vi "FeedBack Chanel.vi"(0 "Test Name":string, 5 "Channels (Int)":i32[](array[numeric]), 7 "FeedBack Channel":string[](array[string])=["fgdgfvcbc", "vnfhgjkn", "21354682"], 9 "Wait/Poll (ms)":u32, 11 "Parameter":u8) -> (4 "Out":i32, 6 "Array":bool[](array[boolean]), 10 "Exit":bool, 12 "Input Status":bool[](array[boolean]), 13 "Channel No":i32[](array[numeric]))   [LabVIEW 2015]
uses:
  Galobal variable_TI.vi
  Project Setup/Globle Variable/GR_Servo.vi
panel:
  out "Result Lvdt":T1
  out "Pokayoka Result":cluster{"Sensor Name":string, "Boolean":bool}[](array[cluster])
  out "output array":bool[](array[boolean])
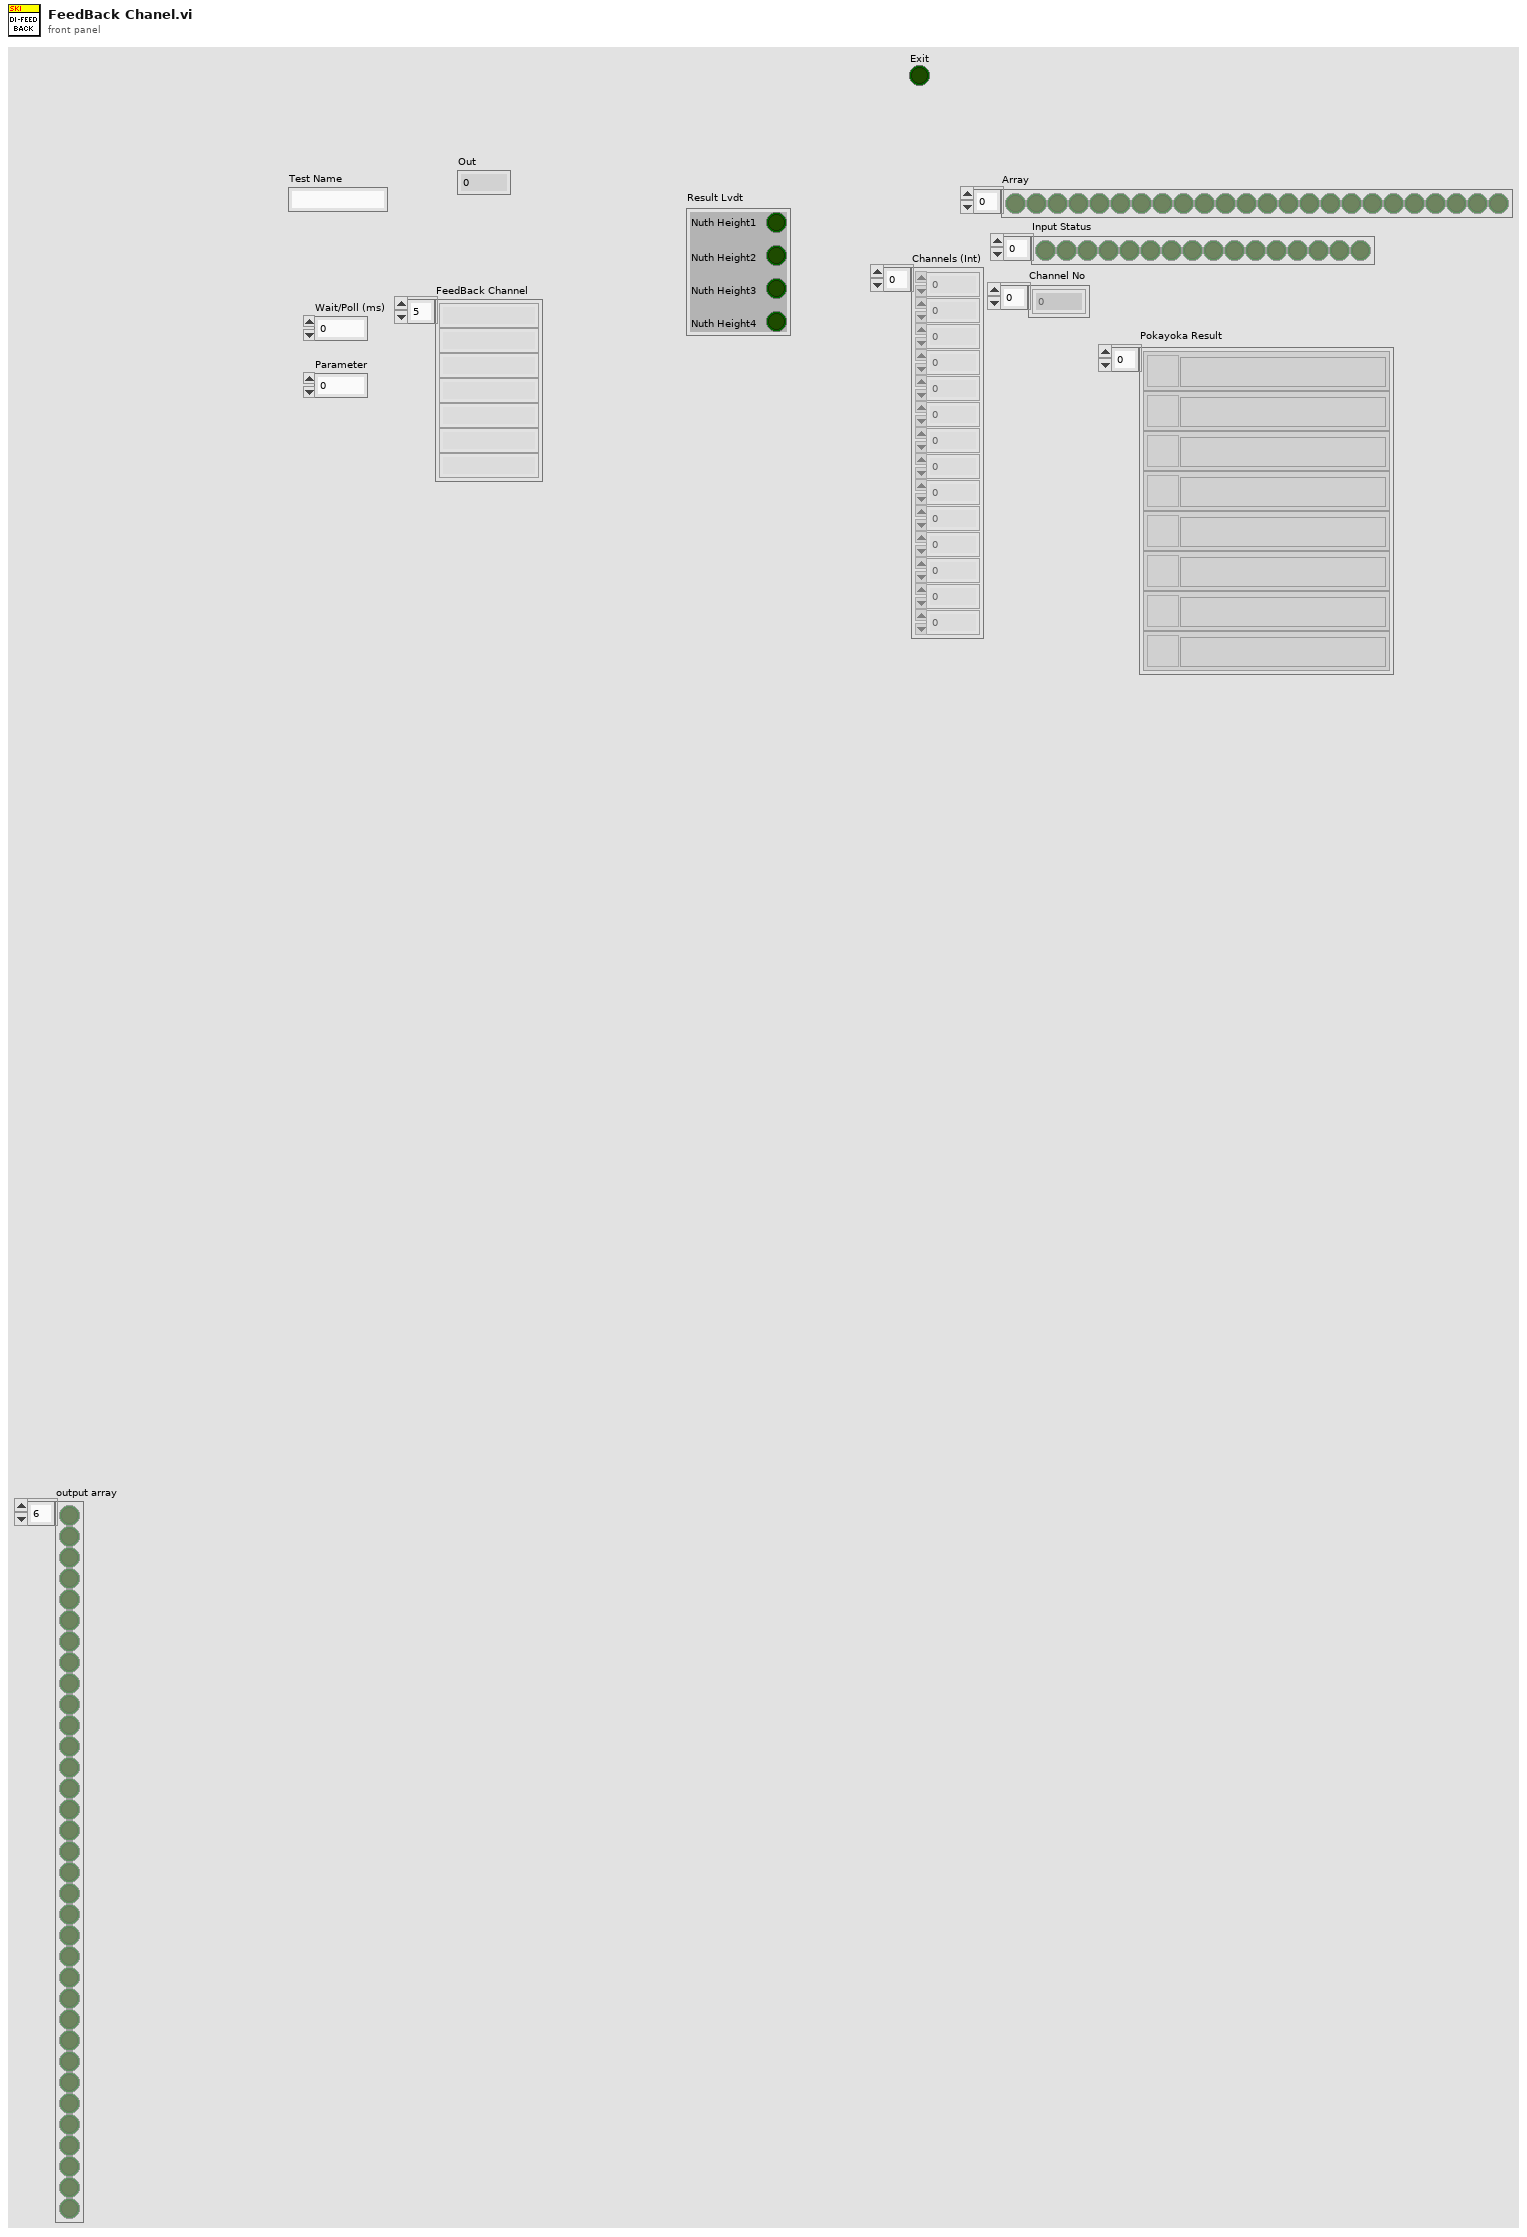
[diagram p1: front panel]
types:
  T1 = cluster{"Nuth Height1":bool, "Nuth Height2":bool, "Nuth Height3":bool, "Nuth Height4":bool}
  T2 = cluster{"LVDT1Max(mm) AI0":dbl, "LVDT1Min (mm)AI0":dbl, "LVDT2Max(mm) AI1":dbl, "LVDT2Min(mm) AI1":dbl, "LVDT3Max(mm) AI2":dbl, "LVDT3Min(mm) AI2":dbl, "LVDT4Max(mm) AI3":dbl, "LVDT4Min(mm) AI3":dbl, "Model":string, "MIC Code":string}
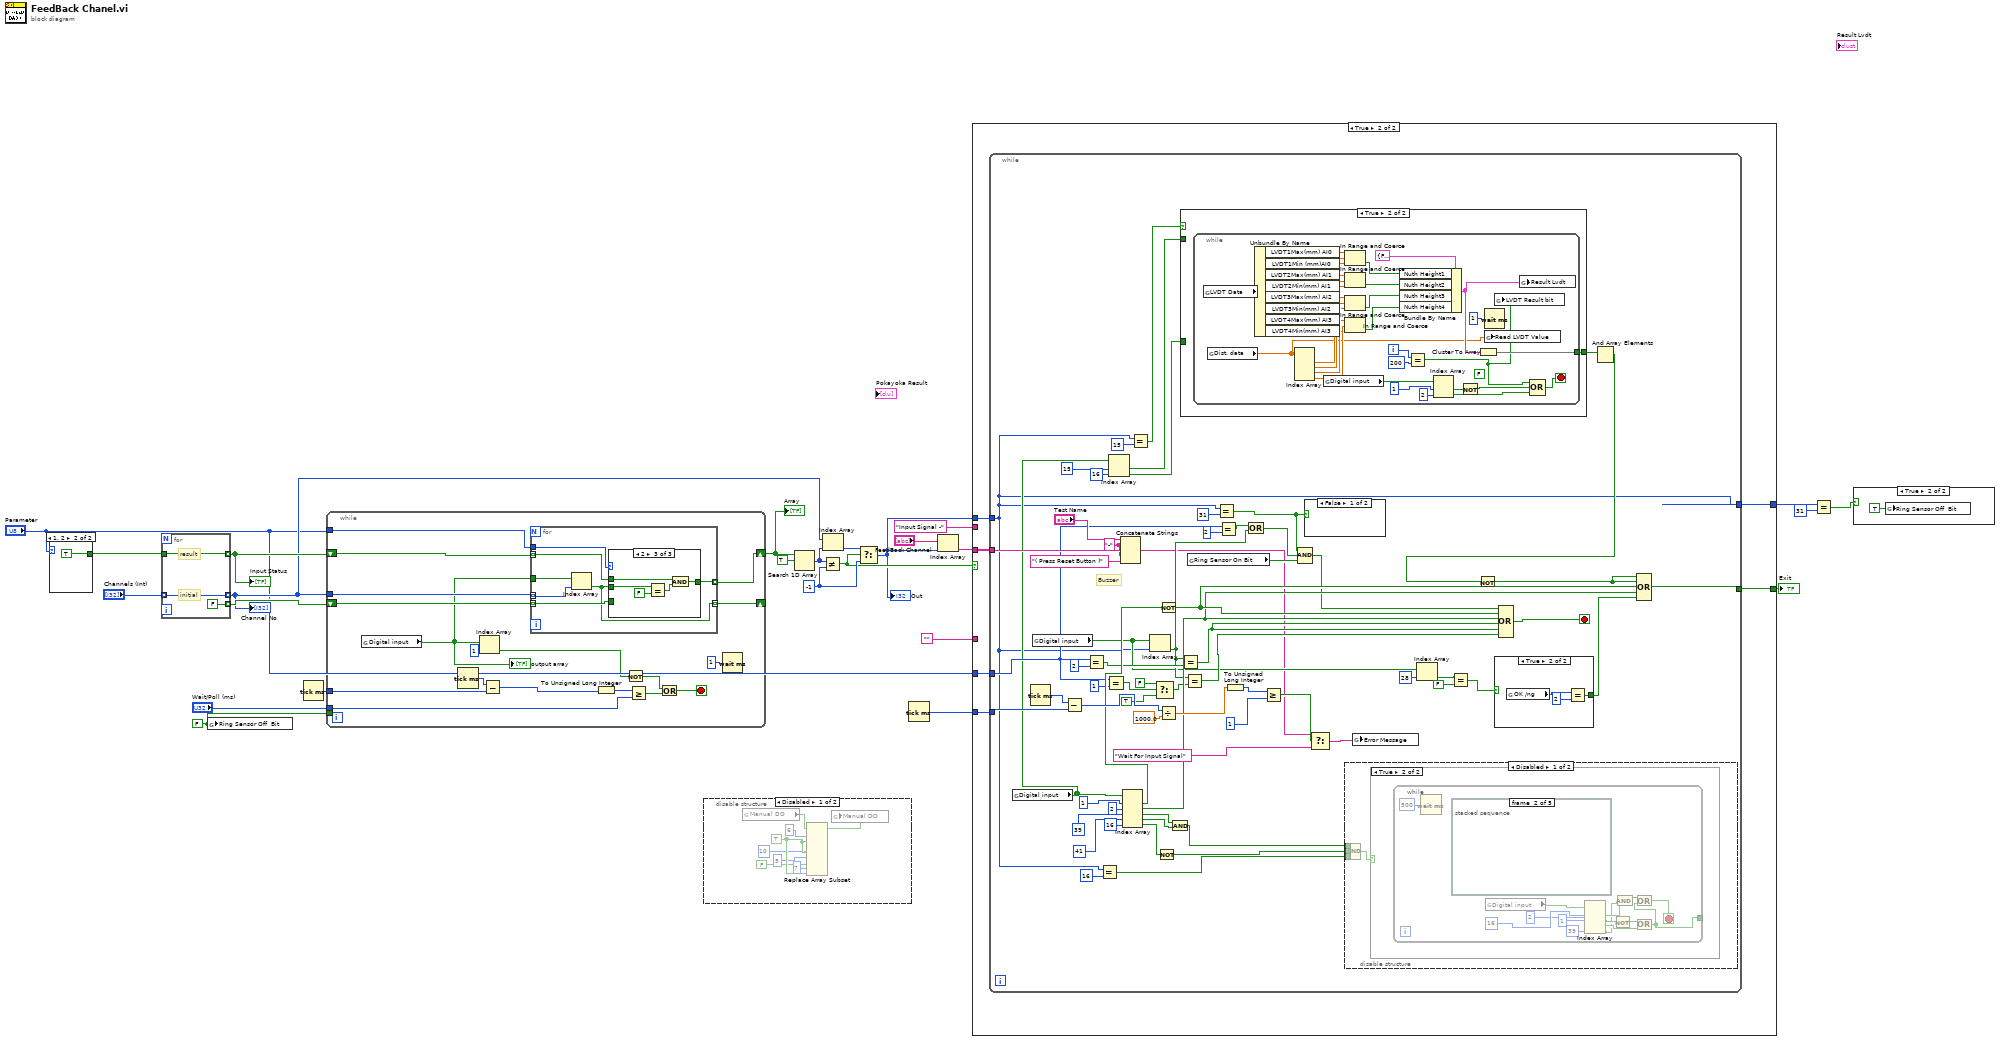
[diagram p0: block diagram]
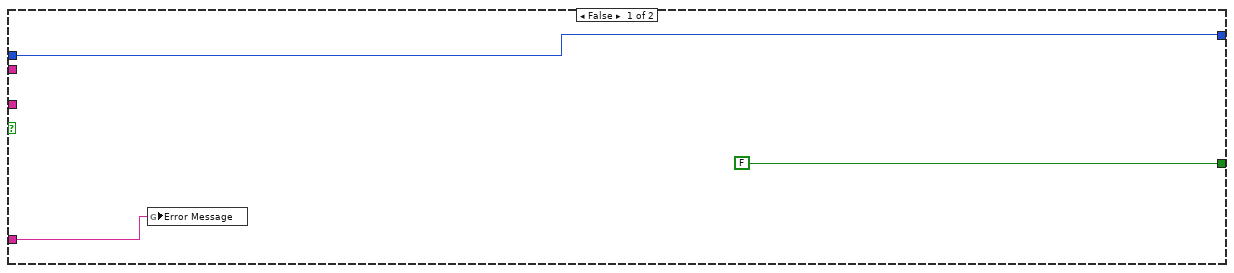
[diagram p4: hidden frame]
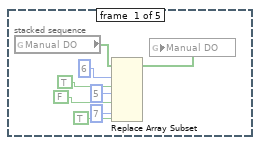
[diagram p6: hidden frame]
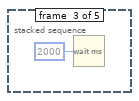
[diagram p7: hidden frame]
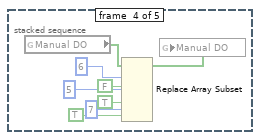
[diagram p8: hidden frame]
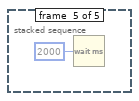
[diagram p9: hidden frame]
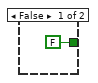
[diagram p11: hidden frame]
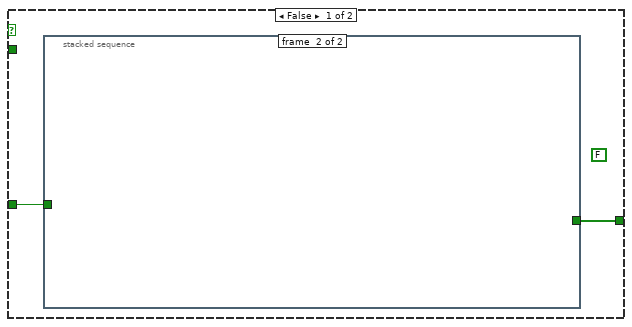
[diagram p12: hidden frame]
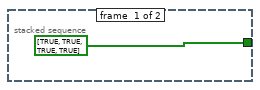
[diagram p13: hidden frame]
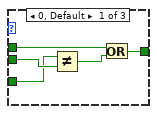
[diagram p15: hidden frame]
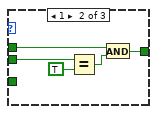
[diagram p16: hidden frame]
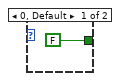
[diagram p17: hidden frame]
diagram:
  w1 = FALSE ("Ring Sensor Off  Bit")
  w25 = -1 ("y")
  n1 = case shown="1, 2" "Parameter" {
    tunnel: [FALSE TRUE] -> w16
    frame 0, Default {
    }
    frame 1, 2 {
    }
  }
  n2 = for {
    tunnel: [w30] -> w11 mode=indexing
    tunnel: w16 -> [w30]
    tunnel: "Channels (Int)" -> [w29] mode=indexing
    tunnel: [w29] -> w10 mode=indexing
    tunnel: [FALSE] -> w20 mode=indexing
    # "result"
    # "initial"
  }
  "Input Status" <- w11
  "Channel No" <- w10
  n3 = global write "Galobal variable_TI.vi" "Ring Sensor Off  Bit"(w1) -> ()
  n4 = Tick Count (ms)() -> (millisecond timer value=w19:u32)
  n5 = while {
    tunnel: "Wait/Poll (ms)" -> [w36]
    tunnel: w19 -> [w47]
    tunnel: w10 -> [w45]
    tunnel: "Parameter" -> [w44]
    shift-right: [w43] -> w22
    shift-left: w11 -> [w41]
    shift-right: [w42] -> _
    shift-left: w20 -> [w40]
    tunnel: w1 -> [_]
    stop <- w38 stop-if-true
    n6 = global read "Galobal variable_TI.vi" "Digital input"() -> (w32:bool[])
    "output array" <- w32
    n7 = Tick Count (ms)() -> (millisecond timer value=w48:u32)
    n8 = Index Array(array=w32, index=1) -> (element=w34:bool)
    n9 = Subtract(x=w48, y=w47) -> (x-y=w31:u32)
    n10 = for {
      tunnel: w40 -> [w50] mode=indexing
      tunnel: w41 -> [w52] mode=indexing
      tunnel: w32 -> [w55]
      tunnel: w45 -> [w54] mode=indexing
      tunnel: w44 -> [w53]
      tunnel: [w51] -> w43 mode=indexing
      tunnel: [w49] -> w42 mode=indexing
      n11 = Index Array(array=w55, index=w54) -> (element=w49:bool)
      n12 = case shown="2" w53 {
        tunnel: w49 -> [w60 w63 w70]
        tunnel: w52 -> [w58 w62 w67]
        tunnel: [w56 w61 w66] -> w51
        tunnel: w50 -> [w59 _ _]
        frame 0, Default {
          n13 = Not Equal?(x=w59, y=w60) -> (x != y?=w57:bool)
          n14 = Or(x=w58, y=w57) -> (x .or. y?=w56:bool)
        }
        frame 1 {
          n15 = Equal?(x=w63, y=TRUE) -> (x = y?=w64:bool)
          n16 = And(x=w62, y=w64) -> (x .and. y?=w61:bool)
        }
        frame 2 {
          n17 = Equal?(x=w70, y=FALSE) -> (x = y?=w68:bool)
          n18 = And(x=w67, y=w68) -> (x .and. y?=w66:bool)
        }
      }
    }
    n19 = To Unsigned Long Integer(number=w31) -> (unsigned 32bit integer=w46:u32)
    n20 = Not(x=w34) -> (.not. x?=w35:bool)
    n21 = Greater Or Equal?(x=w46, y=w36) -> (x >= y?=w39:bool)
    n22 = Or(x=w35, y=w39) -> (x .or. y?=w38:bool)
    n23 = Wait (ms)(milliseconds to wait=u32 1) -> ()  [unwired: 1 out]
  }
  "Array" <- w22
  n24 = disable-structure shown="Disabled" {
    frame Disabled {
      w77 = TRUE ("new element/subarray")
      n25 = global read "Galobal variable_TI.vi" "Manual DO"() -> (w72:bool[])
      n26 = Replace Array Subset(array=w72, new element #1=w77, index #1=6 ("index"), new element #2=w77, index #2=10 ("index"), new element #3=FALSE ("new element/subarray"), index #3=5 ("index"), new element #4=w77, index #4=7 ("index")) -> (w73:bool[])
      n27 = global write "Galobal variable_TI.vi" "Manual DO"(w73) -> ()
    }
    frame Enabled {
    }
  }
  n28 = Search 1D Array(1D array=w22, element=TRUE) -> (index of element=w23:i32)  [unwired: 1 in]
  n29 = Not Equal?(x=w23, y=w25) -> (x != y?=w15:bool)
  n30 = Index Array(array=w10, index=w23) -> (element=w24:i32)
  n31 = Select(t=w24, s=w15, f=w25) -> (s? t:f=w14:i32)
  "Out" <- w14
  n32 = Tick Count (ms)() -> (millisecond timer value=w8:u32)
  n33 = Index Array(array="FeedBack Channel", index=w14) -> (element=w13:string)
  n34 = case shown="True" w15 {
    tunnel: w14 -> [w79 w86]
    tunnel: w13 -> [_ w87]
    tunnel: "Input Signal -" ("string") -> [_ _]
    tunnel: w8 -> [_ w85]
    tunnel: "" -> [w81 _]
    tunnel: [FALSE w84] -> w5
    tunnel: "Parameter" -> [_ w83]
    tunnel: [w79 w82] -> w3
    frame False {
      n35 = global write "GR_Servo.vi" "Error Message"(w81) -> ()
    }
    frame True {
      n36 = while {
        tunnel: w87 -> [w154]
        tunnel: w86 -> [w102]
        tunnel: w85 -> [w146]
        tunnel: [w135] -> w84
        tunnel: w83 -> [w123]
        tunnel: [w102] -> w82
        stop <- w152 stop-if-true
        w150 = "-" ("string")
        # "Buzzer"
        n37 = global read "Galobal variable_TI.vi" "Digital input"() -> (w114:bool[])
        n38 = Tick Count (ms)() -> (millisecond timer value=w149:u32)
        n39 = global read "Galobal variable_TI.vi" "Digital input"() -> (w109:bool[])
        n40 = Subtract(x=w149, y=w146) -> (x-y=w148:u32)
        n41 = Equal?(x=w123, y=u8 2) -> (x = y?=w132:bool)
        n42 = Equal?(x=w102, y=16) -> (x = y?=w89:bool)
        n43 = Equal?(x=w123, y=u8 1) -> (x = y?=w130:bool)
        n44 = Index Array(array=w114, index #1=15 ("index"), index #2=16 ("index")) -> (element #1=w112:bool, element #2=w100:bool)
        n45 = Concatenate Strings("Test Name", w150, w154, w150, "( Press Reset Button )" ("string")) -> (w91:string)
        n46 = Index Array(array=w114, index #1=1 ("index"), index #2=2 ("index"), index #3=39 ("index"), index #4=41 ("index"), index #5=16 ("index")) -> (element #1=w139:bool, element #2=w136:bool, element #3=w96:bool, element #4=w95:bool, element #5=w90:bool)
        n47 = Equal?(x=w102, y=15) -> (x = y?=w115:bool)
        n48 = Index Array(array=w109, index=w102) -> (element=w121:bool)
        n49 = Select(t=FALSE, s=w130, f=TRUE) -> (s? t:f=w127:bool)
        n50 = Not(x=w90) -> (.not. x?=w92:bool)
        n51 = Not(x=w139) -> (.not. x?=w137:bool)
        n52 = Divide(x=w148, y=1000.0) -> (x/y=w144:dbl)
        n53 = Compound Arithmetic op=AND(w96, w95) -> (w93:bool)
        n54 = case shown="True" w115 {
          tunnel: w112 -> [_ _]
          tunnel: [w196 w198] -> w111
          tunnel: w100 -> [w195 _]
          frame False {
            (unwired) FALSE ("LVDT Result bit")
            n55 = stacked-sequence {
              tunnel: [bool[] [TRUE, TRUE, TRUE, TRUE] ("Result Lvdt") _] -> w196
              tunnel: w195 -> [_ _]
              frame #0 {
              }
              frame #1 {
              }
            }
          }
          frame True {
            n56 = while {
              tunnel: [w200] -> w198
              i -> [w230]
              stop <- w202 stop-if-true
              (unwired) FALSE
              n57 = global read "Galobal variable_TI.vi" "LVDT Data"() -> (w210:T2)
              n58 = global read "Galobal variable_TI.vi" "Dist. data"() -> (w201:dbl[])
              n59 = Unbundle By Name(w210) -> ("LVDT1Max(mm) AI0"=w211:dbl, "LVDT1Min (mm)AI0"=w212:dbl, "LVDT2Max(mm) AI1"=w213:dbl, "LVDT2Min(mm) AI1"=w219:dbl, "LVDT3Max(mm) AI2"=w214:dbl, "LVDT3Min(mm) AI2"=w215:dbl, "LVDT4Max(mm) AI3"=w216:dbl, "LVDT4Min(mm) AI3"=w217:dbl)
              n60 = Index Array(array=w201) -> (element #1=w218:dbl, element #2=w220:dbl, element #3=w221:dbl, element #4=w222:dbl)  [unwired: 4 in]
              n61 = global read "Galobal variable_TI.vi" "Digital input"() -> (w206:bool[])
              n62 = In Range and Coerce(upper limit=w211, x=w218, lower limit=w212) -> (In Range?=w224:bool)  [unwired: 1 out]
              n63 = In Range and Coerce(upper limit=w213, x=w220, lower limit=w219) -> (In Range?=w225:bool)  [unwired: 1 out]
              n64 = In Range and Coerce(upper limit=w214, x=w221, lower limit=w215) -> (In Range?=w226:bool)  [unwired: 1 out]
              n65 = In Range and Coerce(upper limit=w216, x=w222, lower limit=w217) -> (In Range?=w227:bool)  [unwired: 1 out]
              n66 = Bundle By Name(cluster=T1 {"Nuth Height1"=FALSE, "Nuth Height2"=FALSE, "Nuth Height3"=FALSE, "Nuth Height4"=FALSE} ("Result Lvdt"), "Nuth Height1"=w224, "Nuth Height2"=w225, "Nuth Height3"=w226, "Nuth Height4"=w227) -> (w209:T1)
              n67 = Equal?(x=w230, y=200) -> (x = y?=w199:bool)
              n68 = Index Array(array=w206, index #1=1 ("index"), index #2=2 ("index")) -> (element #1=w205:bool, element #2=w203:bool)
              n69 = Not(x=w205) -> (.not. x?=w204:bool)
              n70 = Cluster To Array(cluster=w209) -> (array=w200:bool[])
              n71 = Wait (ms)(milliseconds to wait=u32 1) -> ()  [unwired: 1 out]
              n72 = global write "Galobal variable_TI.vi" "Read LVDT Value"(w201) -> ()
              n73 = global write "Galobal variable_TI.vi" "LVDT Result bit"(w199) -> ()
              n74 = global write "Galobal variable_TI.vi" "Result Lvdt"(w209) -> ()
              n75 = Compound Arithmetic op=OR(w199, w204, w203) -> (w202:bool)
            }
          }
        }
        n76 = Equal?(x=w121, y=w132) -> (x = y?=w126:bool)
        n77 = Equal?(x=w121, y=w127) -> (x = y?=w131:bool)
        n78 = global read "Galobal variable_TI.vi" "Ring Sensor On Bit"() -> (w118:bool)
        n79 = Equal?(x=w102, y=31) -> (x = y?=w119:bool)
        n80 = Equal?(x=w123, y=2) -> (x = y?=w122:bool)
        n81 = To Unsigned Long Integer(number=w144) -> (unsigned 32bit integer=w88:u32)
        n82 = Compound Arithmetic op=OR(w122, w121) -> (w120:bool)
        n83 = Greater Or Equal?(x=w88, y=u32 1) -> (x >= y?=w143:bool)
        n84 = Compound Arithmetic op=AND(w119, w120, w118) -> (w117:bool)
        n85 = case shown="False" w119 {
          frame False {
          }
          frame True {
          }
        }
        n86 = Select(t=w91, s=w143, f="Wait For Input Signal") -> (s? t:f=w141:string)
        n87 = disable-structure shown="Disabled" {
          disable-tunnel: w93 -> [w158 _]
          disable-tunnel: w92 -> [w156 _]
          disable-tunnel: w89 -> [w155 _]
          frame Disabled {
            n88 = Compound Arithmetic op=AND(w158, w156, w155) -> (w157:bool)
            n89 = case shown="True" w157 {
              frame False {
              }
              frame True {
                n90 = while {
                  tunnel: [w163] -> _
                  stop <- w164 stop-if-true
                  n91 = Wait (ms)(milliseconds to wait=u32 500) -> ()  [unwired: 1 out]
                  n92 = stacked-sequence {
                    frame #0 {
                      n93 = global read "Galobal variable_TI.vi" "Manual DO"() -> (w178:bool[])
                      n94 = Replace Array Subset(array=w178, new element #1=TRUE ("new element/subarray"), index #1=6 ("index"), new element #2=FALSE ("new element/subarray"), index #2=5 ("index"), new element #3=TRUE ("new element/subarray"), index #3=7 ("index")) -> (w177:bool[])
                      n95 = global write "Galobal variable_TI.vi" "Manual DO"(w177) -> ()
                    }
                    frame #1 {
                    }
                    frame #2 {
                      n96 = Wait (ms)(milliseconds to wait=u32 2000) -> ()  [unwired: 1 out]
                    }
                    frame #3 {
                      n97 = global read "Galobal variable_TI.vi" "Manual DO"() -> (w187:bool[])
                      n98 = Replace Array Subset(array=w187, new element #1=FALSE ("new element/subarray"), index #1=6 ("index"), new element #2=TRUE ("new element/subarray"), index #2=5 ("index"), new element #3=TRUE ("new element/subarray"), index #3=7 ("index")) -> (w186:bool[])
                      n99 = global write "Galobal variable_TI.vi" "Manual DO"(w186) -> ()
                    }
                    frame #4 {
                      n100 = Wait (ms)(milliseconds to wait=u32 2000) -> ()  [unwired: 1 out]
                    }
                  }
                  n101 = global read "Galobal variable_TI.vi" "Digital input"() -> (w172:bool[])
                  n102 = Index Array(array=w172, index #1=16 ("index"), index #2=1 ("index"), index #3=2 ("index"), index #4=39 ("index")) -> (element #1=w165:bool, element #2=w168:bool, element #3=w166:bool, element #4=w159:bool)
                  n103 = Not(x=w168) -> (.not. x?=w167:bool)
                  n104 = And(x=w165, y=w159) -> (x .and. y?=w160:bool)
                  n105 = Or(x=w167, y=w166) -> (x .or. y?=w163:bool)
                  n106 = Or(x=w160, y=w163) -> (x .or. y?=w164:bool)
                }
              }
            }
          }
          frame Enabled {
          }
        }
        n107 = global write "GR_Servo.vi" "Error Message"(w141) -> ()
        n108 = Index Array(array=w109, index=28) -> (element=w107:bool)
        n109 = Equal?(x=w107, y=FALSE) -> (x = y?=w105:bool)
        n110 = case shown="True" w105 {
          tunnel: [FALSE w192] -> w104
          frame False {
          }
          frame True {
            n111 = global read "Galobal variable_TI.vi" "OK /ng"() -> (w194:i32)
            n112 = Equal?(x=w194, y=2) -> (x = y?=w192:bool)
          }
        }
        n113 = Compound Arithmetic op=OR(w117, w137, w136, w126, w126, w131) -> (w152:bool)
        n114 = And Array Elements(Boolean array=w111) -> (logical AND=w110:bool)
        n115 = Not(x=w110) -> (.not. x?=w99:bool)
        n116 = Compound Arithmetic op=OR(w99, w99, w137, w136, w104) -> (w135:bool)
      }
    }
  }
  "Exit" <- w5
  n117 = Equal?(x=w3, y=31) -> (x = y?=w2:bool)
  n118 = case shown="True" w2 {
    frame False {
    }
    frame True {
      n119 = global write "Galobal variable_TI.vi" "Ring Sensor Off  Bit"(TRUE ("Ring Sensor Off  Bit")) -> ()
    }
  }
